vi "main.vi"() -> ()   [LabVIEW 2023]
uses:
  #typedef_state.ctl
  #typdef_data.ctl
panel:
  in  "Reset":bool
  in  "0":bool caption="Blank Button 6"
  in  "9":bool caption="Blank Button"
  in  "8":bool caption="Blank Button 5"
  in  "7":bool caption="Blank Button 4"
  in  "6":bool caption="Blank Button 3"
  in  "5":bool caption="Blank Button 2"
  in  "4":bool caption="Blank Button"
  in  "3":bool caption="Blank Button"
  in  "2":bool caption="Blank Button"
  in  "1":bool caption="Blank Button"
  in  "Stop Button":bool
  out "Pressed Numbers":string
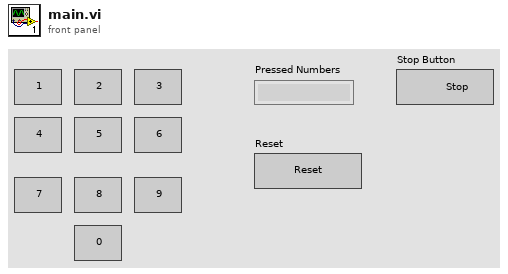
[diagram p1: front panel]
types:
  T1 = typedef "#typedef_state.ctl" = enum16{"Aplication Error", "Exit", "Reset", "9", "8", "7", "6", "5", "4", "3", "2", "1", "0", "Idling", "Inicializing"}
  T2 = typedef "#typdef_data.ctl" = cluster{"String":string}
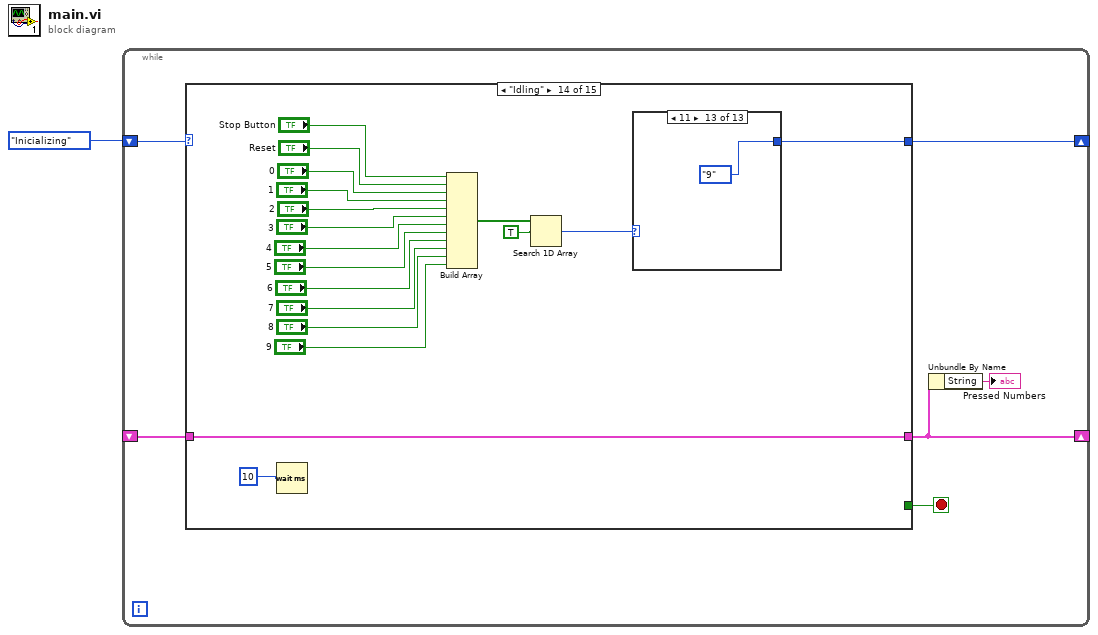
[diagram p0: block diagram]
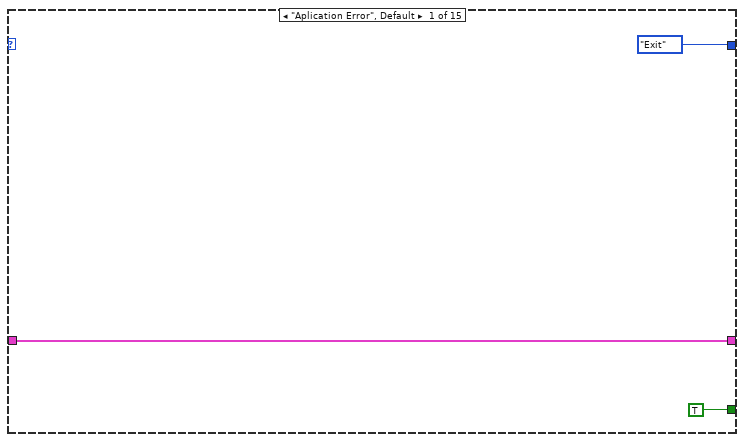
[diagram p2: hidden frame]
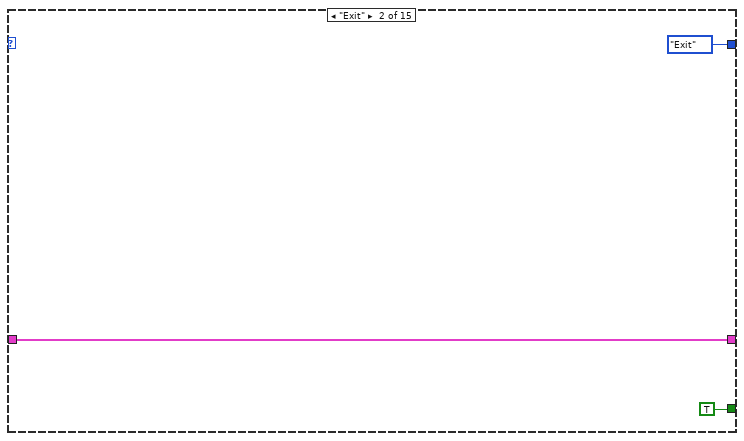
[diagram p3: hidden frame]
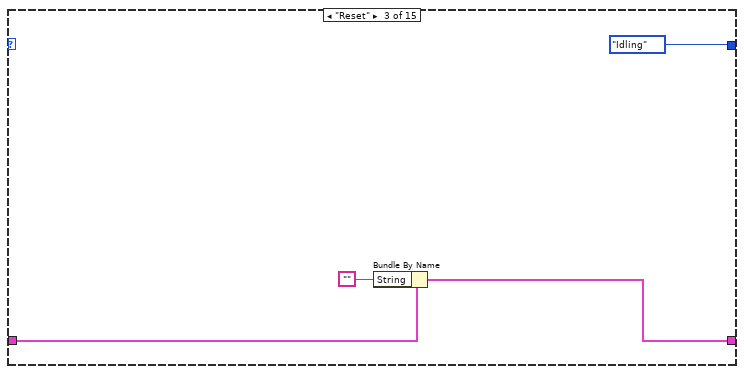
[diagram p4: hidden frame]
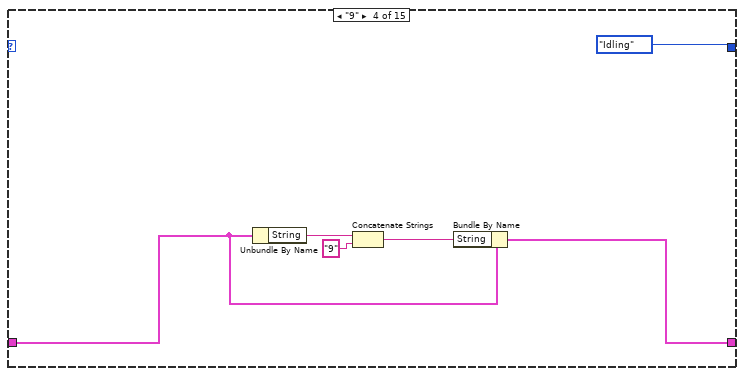
[diagram p5: hidden frame]
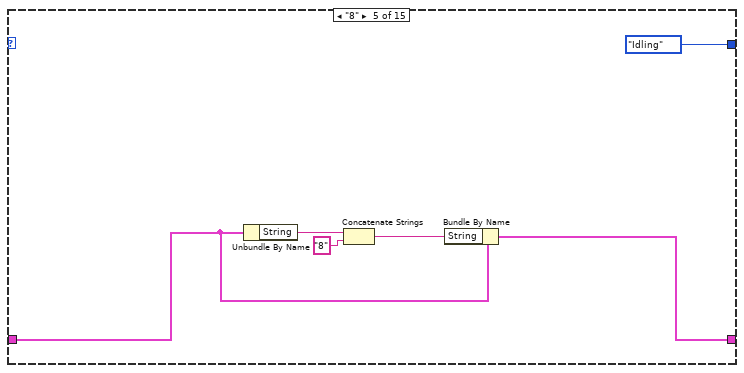
[diagram p6: hidden frame]
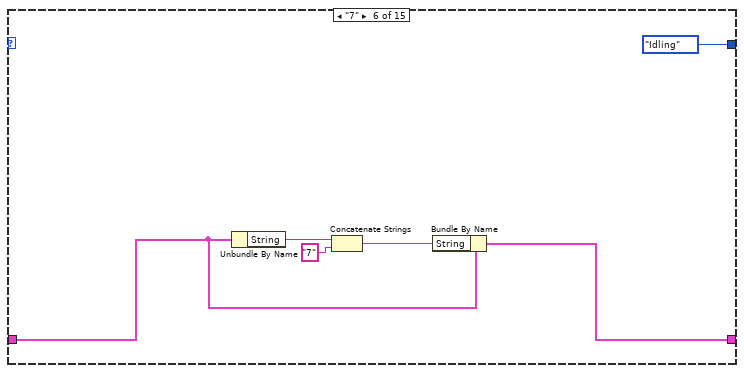
[diagram p7: hidden frame]
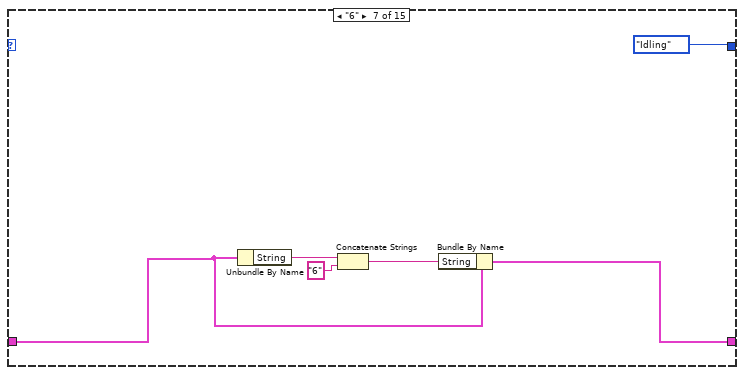
[diagram p8: hidden frame]
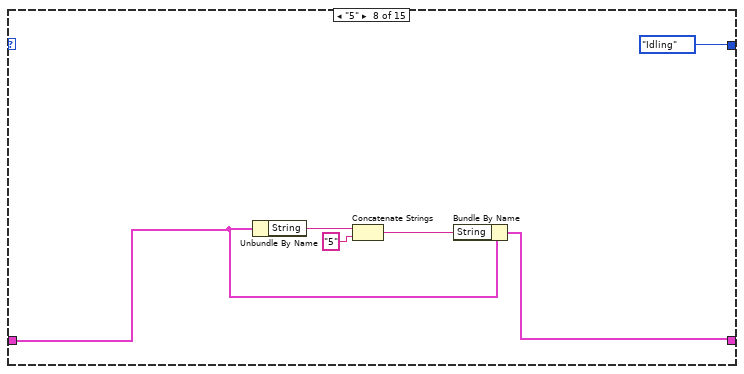
[diagram p9: hidden frame]
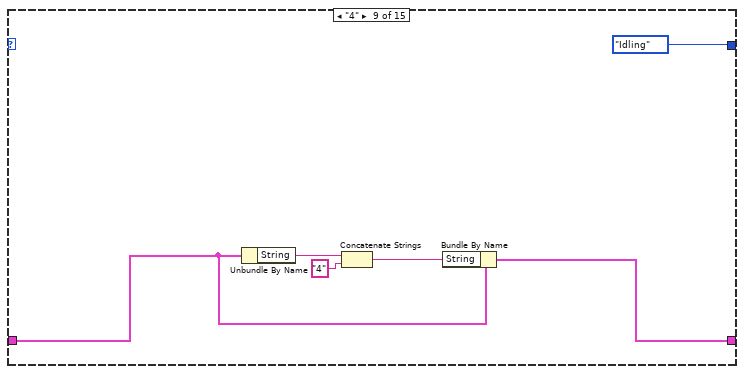
[diagram p10: hidden frame]
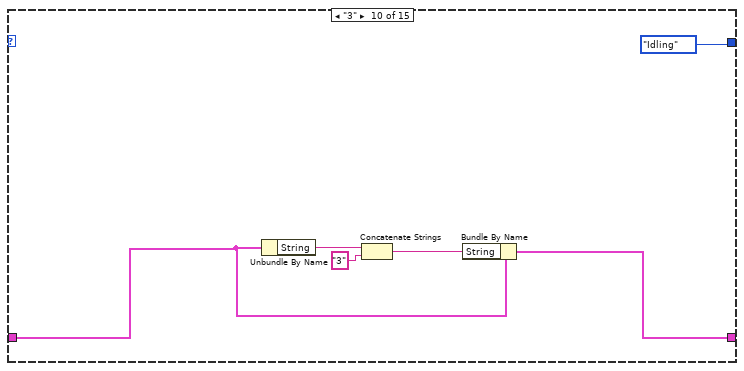
[diagram p11: hidden frame]
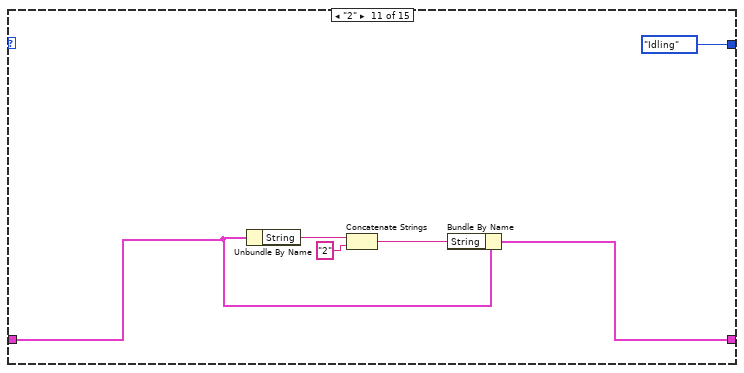
[diagram p12: hidden frame]
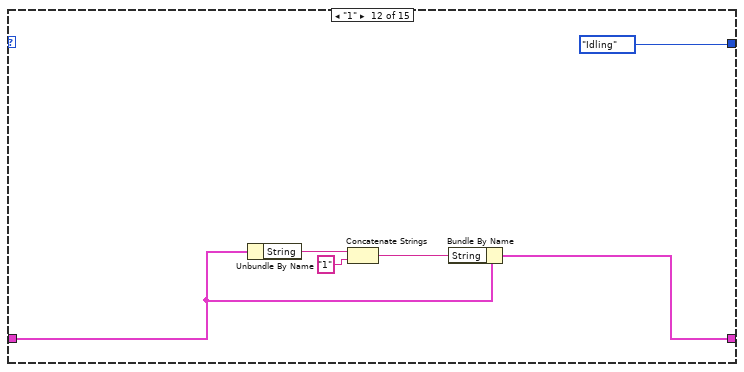
[diagram p13: hidden frame]
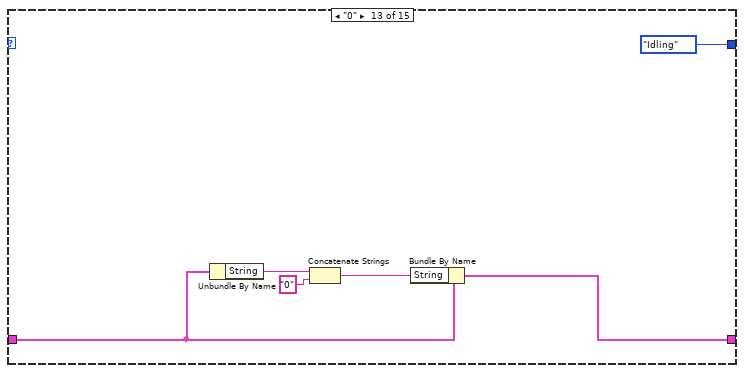
[diagram p14: hidden frame]
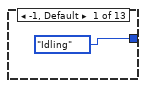
[diagram p15: hidden frame]
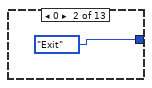
[diagram p16: hidden frame]
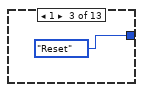
[diagram p17: hidden frame]
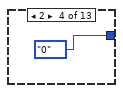
[diagram p18: hidden frame]
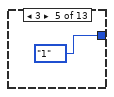
[diagram p19: hidden frame]
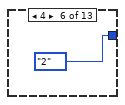
[diagram p20: hidden frame]
diagram:
  n1 = while {
    shift-right: [w6] -> _
    shift-left: #typedef_state."Inicializing" ("State") -> [w7]
    shift-right: [w3] -> _
    shift-left: _ -> [w5]
    stop <- w4 stop-if-true
    n2 = case shown="\"Idling\"" w7 {
      tunnel: [#typedef_state."Exit" ("State") #typedef_state."Exit" ("State") #typedef_state."Idling" ("State") #typedef_state."Idling" ("State") #typedef_state."Idling" ("State") #typedef_state."Idling" ("State") #typedef_state."Idling" ("State") #typedef_state."Idling" ("State") #typedef_state."Idling" ("State") #typedef_state."Idling" ("State") #typedef_state."Idling" ("State") #typedef_state."Idling" ("State") #typedef_state."Idling" ("State") w79 #typedef_state."Idling" ("State")] -> w6
      tunnel: [w10 w13 w15 w19 w25 w30 w36 w42 w48 w54 w61 w67 w73 w95 T2 {"String"=""} ("Data")] -> w3
      tunnel: w5 -> [w10 w13 w16 w20 w26 w31 w37 w43 w49 w55 w62 w68 w77 w95 _]
      tunnel: [TRUE TRUE _ _ _ _ _ _ _ _ _ _ _ _ _] -> w4
      frame "Aplication Error", Default {
      }
      frame "Exit" {
      }
      frame "Reset" {
        n3 = Bundle By Name(cluster=w16, "String"="") -> (w15:T2)
      }
      frame "9" {
        n4 = Unbundle By Name(w20) -> ("String"=w23:string)
        n5 = Concatenate Strings(w23, "9" ("string")) -> (w21:string)
        n6 = Bundle By Name(cluster=w20, "String"=w21) -> (w19:T2)
      }
      frame "8" {
        n7 = Unbundle By Name(w26) -> ("String"=w29:string)
        n8 = Concatenate Strings(w29, "8" ("string")) -> (w27:string)
        n9 = Bundle By Name(cluster=w26, "String"=w27) -> (w25:T2)
      }
      frame "7" {
        n10 = Unbundle By Name(w31) -> ("String"=w35:string)
        n11 = Concatenate Strings(w35, "7" ("string")) -> (w33:string)
        n12 = Bundle By Name(cluster=w31, "String"=w33) -> (w30:T2)
      }
      frame "6" {
        n13 = Unbundle By Name(w37) -> ("String"=w41:string)
        n14 = Concatenate Strings(w41, "6" ("string")) -> (w39:string)
        n15 = Bundle By Name(cluster=w37, "String"=w39) -> (w36:T2)
      }
      frame "5" {
        n16 = Unbundle By Name(w43) -> ("String"=w47:string)
        n17 = Concatenate Strings(w47, "5" ("string")) -> (w45:string)
        n18 = Bundle By Name(cluster=w43, "String"=w45) -> (w42:T2)
      }
      frame "4" {
        n19 = Unbundle By Name(w49) -> ("String"=w53:string)
        n20 = Concatenate Strings(w53, "4" ("string")) -> (w51:string)
        n21 = Bundle By Name(cluster=w49, "String"=w51) -> (w48:T2)
      }
      frame "3" {
        n22 = Unbundle By Name(w55) -> ("String"=w59:string)
        n23 = Concatenate Strings(w59, "3" ("string")) -> (w57:string)
        n24 = Bundle By Name(cluster=w55, "String"=w57) -> (w54:T2)
      }
      frame "2" {
        n25 = Unbundle By Name(w62) -> ("String"=w65:string)
        n26 = Concatenate Strings(w65, "2" ("string")) -> (w63:string)
        n27 = Bundle By Name(cluster=w62, "String"=w63) -> (w61:T2)
      }
      frame "1" {
        n28 = Unbundle By Name(w68) -> ("String"=w71:string)
        n29 = Concatenate Strings(w71, "1" ("string")) -> (w69:string)
        n30 = Bundle By Name(cluster=w68, "String"=w69) -> (w67:T2)
      }
      frame "0" {
        n31 = Unbundle By Name(w77) -> ("String"=w76:string)
        n32 = Concatenate Strings(w76, "0" ("string")) -> (w74:string)
        n33 = Bundle By Name(cluster=w77, "String"=w74) -> (w73:T2)
      }
      frame "Idling" {
        n34 = Wait (ms)(milliseconds to wait=u32 10) -> ()  [unwired: 1 out]
        n35 = Build Array("Stop Button", "Reset", "0", "1", "2", "3", "4", "5", "6", "7", "8", "9") -> (w82:bool[])
        n36 = Search 1D Array(1D array=w82, element=TRUE) -> (index of element=w80:i32)  [unwired: 1 in]
        n37 = case shown="11" w80 {
          tunnel: [#typedef_state."Idling" ("State") #typedef_state."Exit" ("State") #typedef_state."Reset" ("State") #typedef_state."0" ("State") #typedef_state."1" ("State") #typedef_state."2" ("State") #typedef_state."3" ("State") #typedef_state."4" ("State") #typedef_state."5" ("State") #typedef_state."6" ("State") #typedef_state."7" ("State") #typedef_state."8" ("State") #typedef_state."9" ("State")] -> w79
          frame -1, Default {
          }
          frame 0 {
          }
          frame 1 {
          }
          frame 2 {
          }
          frame 3 {
          }
          frame 4 {
          }
          frame 5 {
          }
          frame 6 {
          }
          frame 7 {
          }
          frame 8 {
          }
          frame 9 {
          }
          frame 10 {
          }
          frame 11 {
          }
        }
      }
      frame "Inicializing" {
      }
    }
    n38 = Unbundle By Name(w3) -> ("String"=→"Pressed Numbers":string)
  }
